vi "MAIN_test.vi"() -> ()   [LabVIEW 2016]
uses:
  <vilib>/Utility/file.llb/Write Delimited Spreadsheet (I64).vi
  BT-Android_AE_library/BT-Android_interface.lvlib
panel:
  out "String":string
  in  "Tab Control 2":enum32{"Information", "Console", "验证sd数据"}(tab)
  in  "receive frequence":i32=10
  in  "receive存盘":bool
  in  "receive file path (dialog if empty)":path=path "D:/Data/intan"
  in  "port number":u32=4321
  in  "display file path (dialog if empty)":path=path "D:/Data/intan"
  in  "display存盘":bool
  in  "Right cycle":i32
  in  "Error cycle":i32
  out "Average Error Ratio":dbl format="%#.4f"
  in  "Select IP before run":refnum<visa-resource-name>="192.168.4.1"
  in  "Channels":i32=35
  in  "START CONVERT":bool
  in  "END CONVERT":bool
  in  "校验误码率":bool
  in  "35channel存sd卡":bool
  in  "sd file path":path=path "D:/Data/intan"
  in  "验证sd数据":bool
  in  "Tab Control":enum32{"Page 1", "Page 2"}(tab)
  out "校验Array":u8[](array[numeric])
  out "高8位Array":u8[](array[numeric])
  out "低8位Array":u8[](array[numeric])
  out "display array":u16[](array[numeric])
  out "35通道波形":u16[][](graph)
  out "End Character?":bool
  out "send timeout":bool=TRUE
  out "?":bool=TRUE
  in  "convert?":bool=TRUE
  in  "Send":bool
  in  "Receive":bool=TRUE
  in  "Data Send":string
  out "error out":errorcluster
  in  "Close Com":bool
  in  "timeout (10sec)":u32=10000
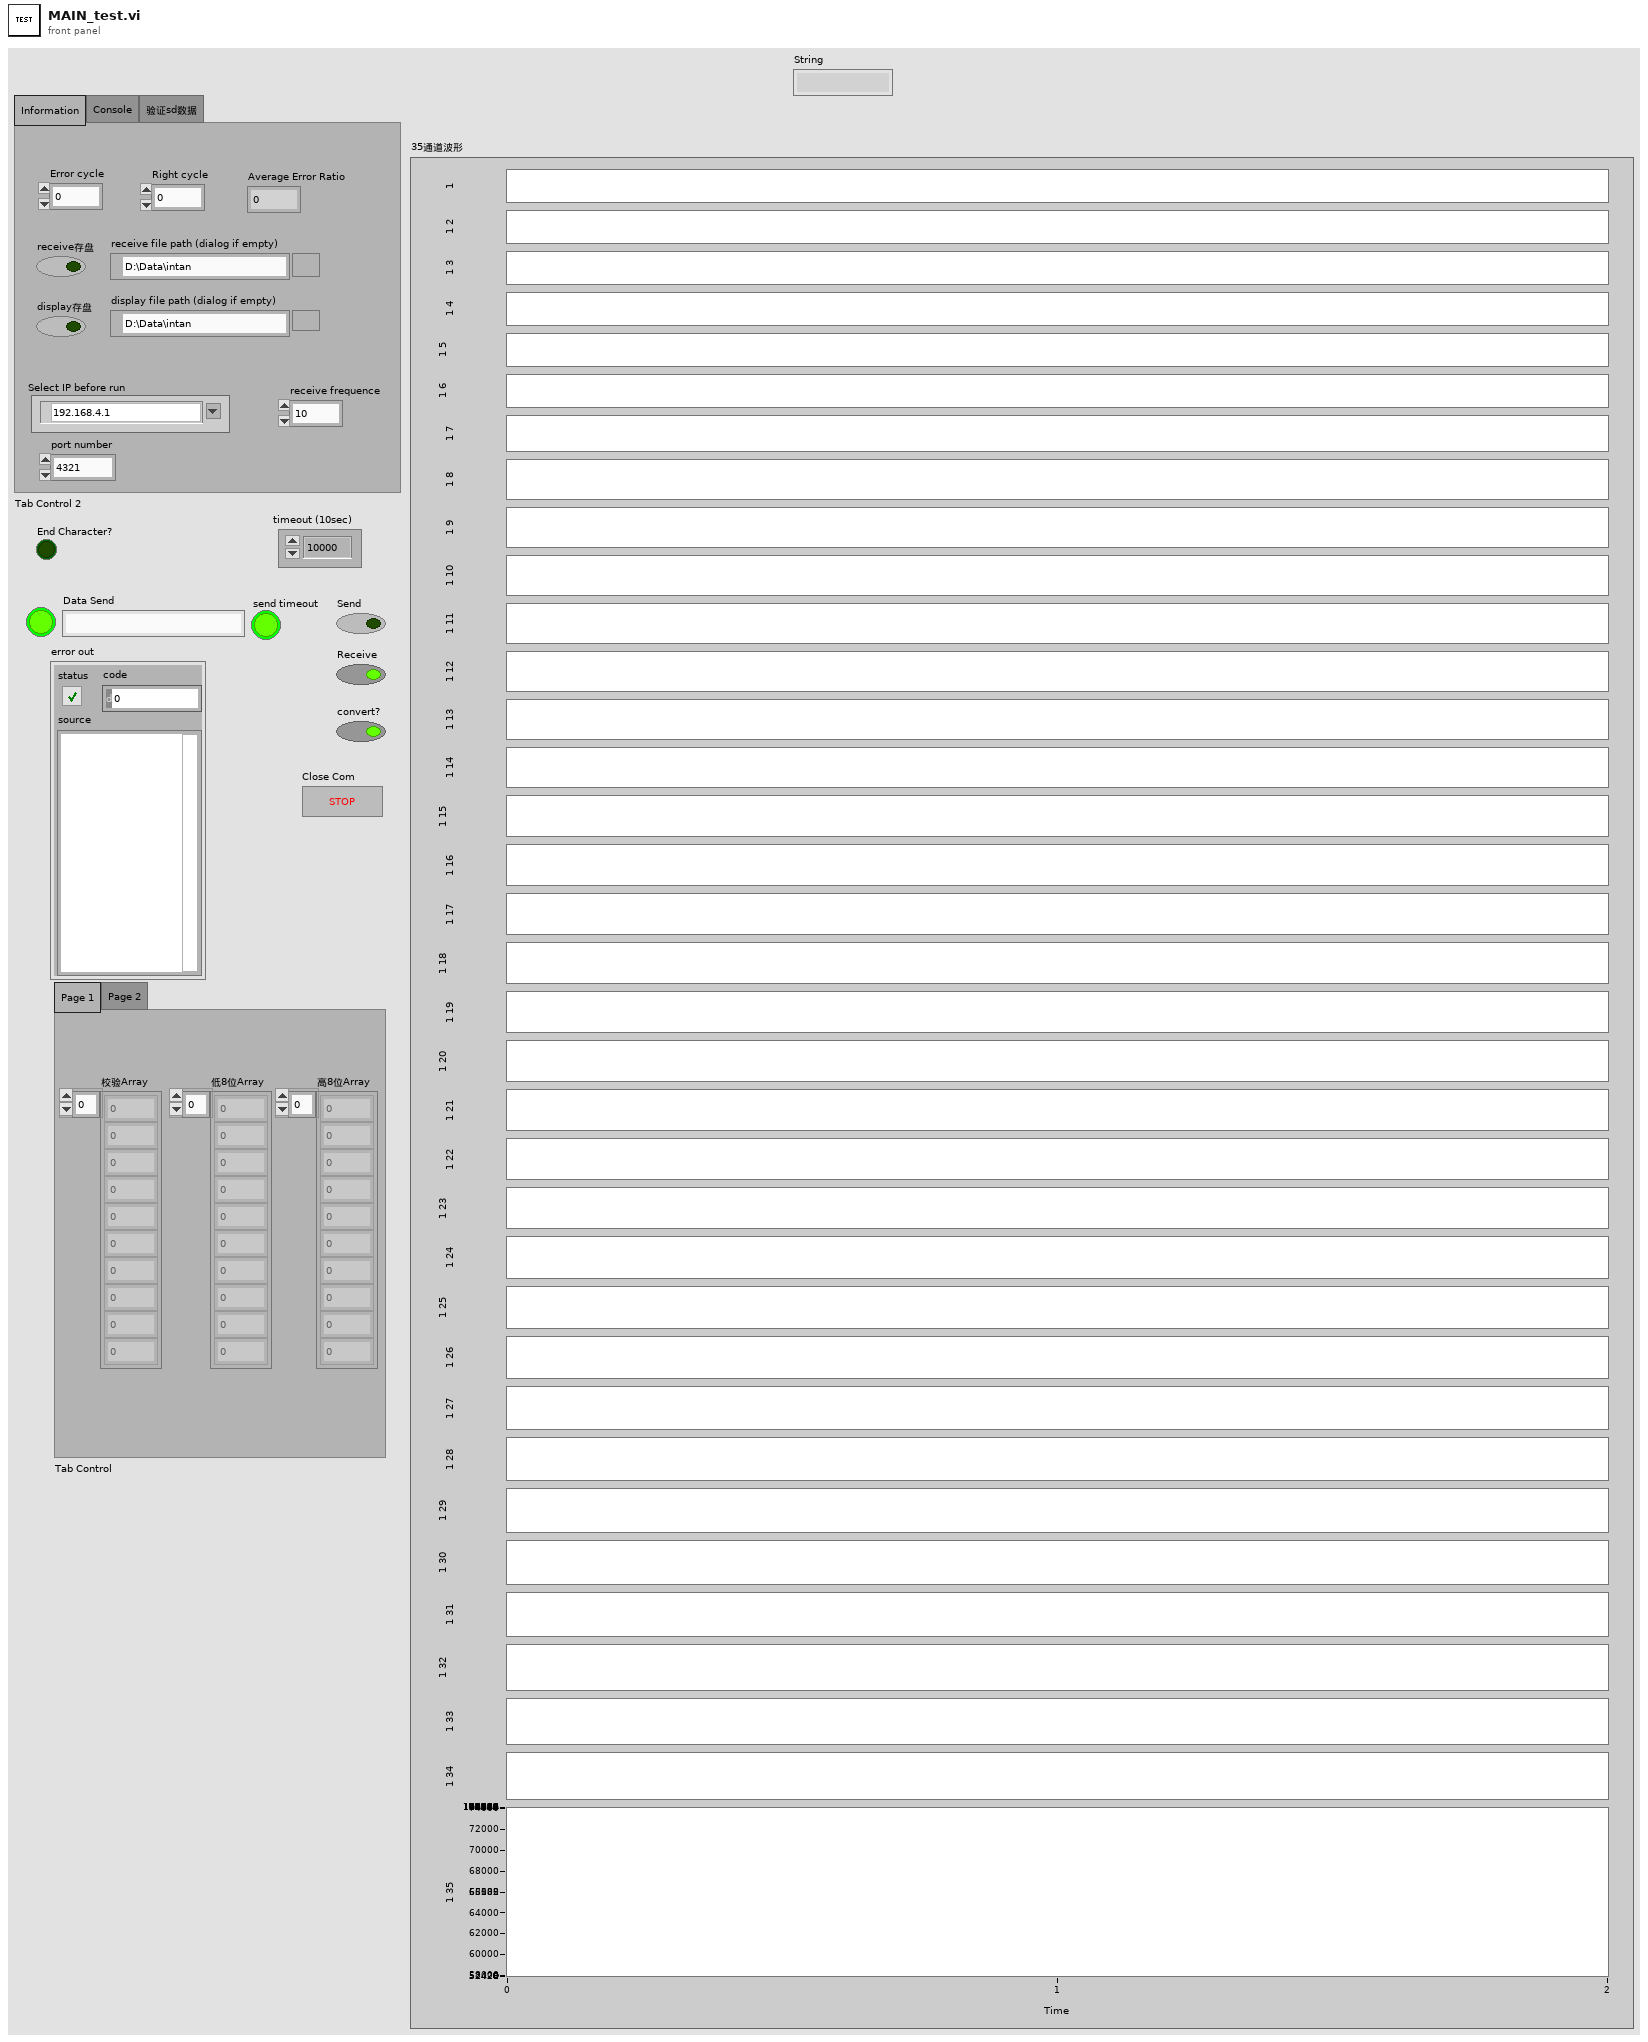
[diagram p1: front panel]
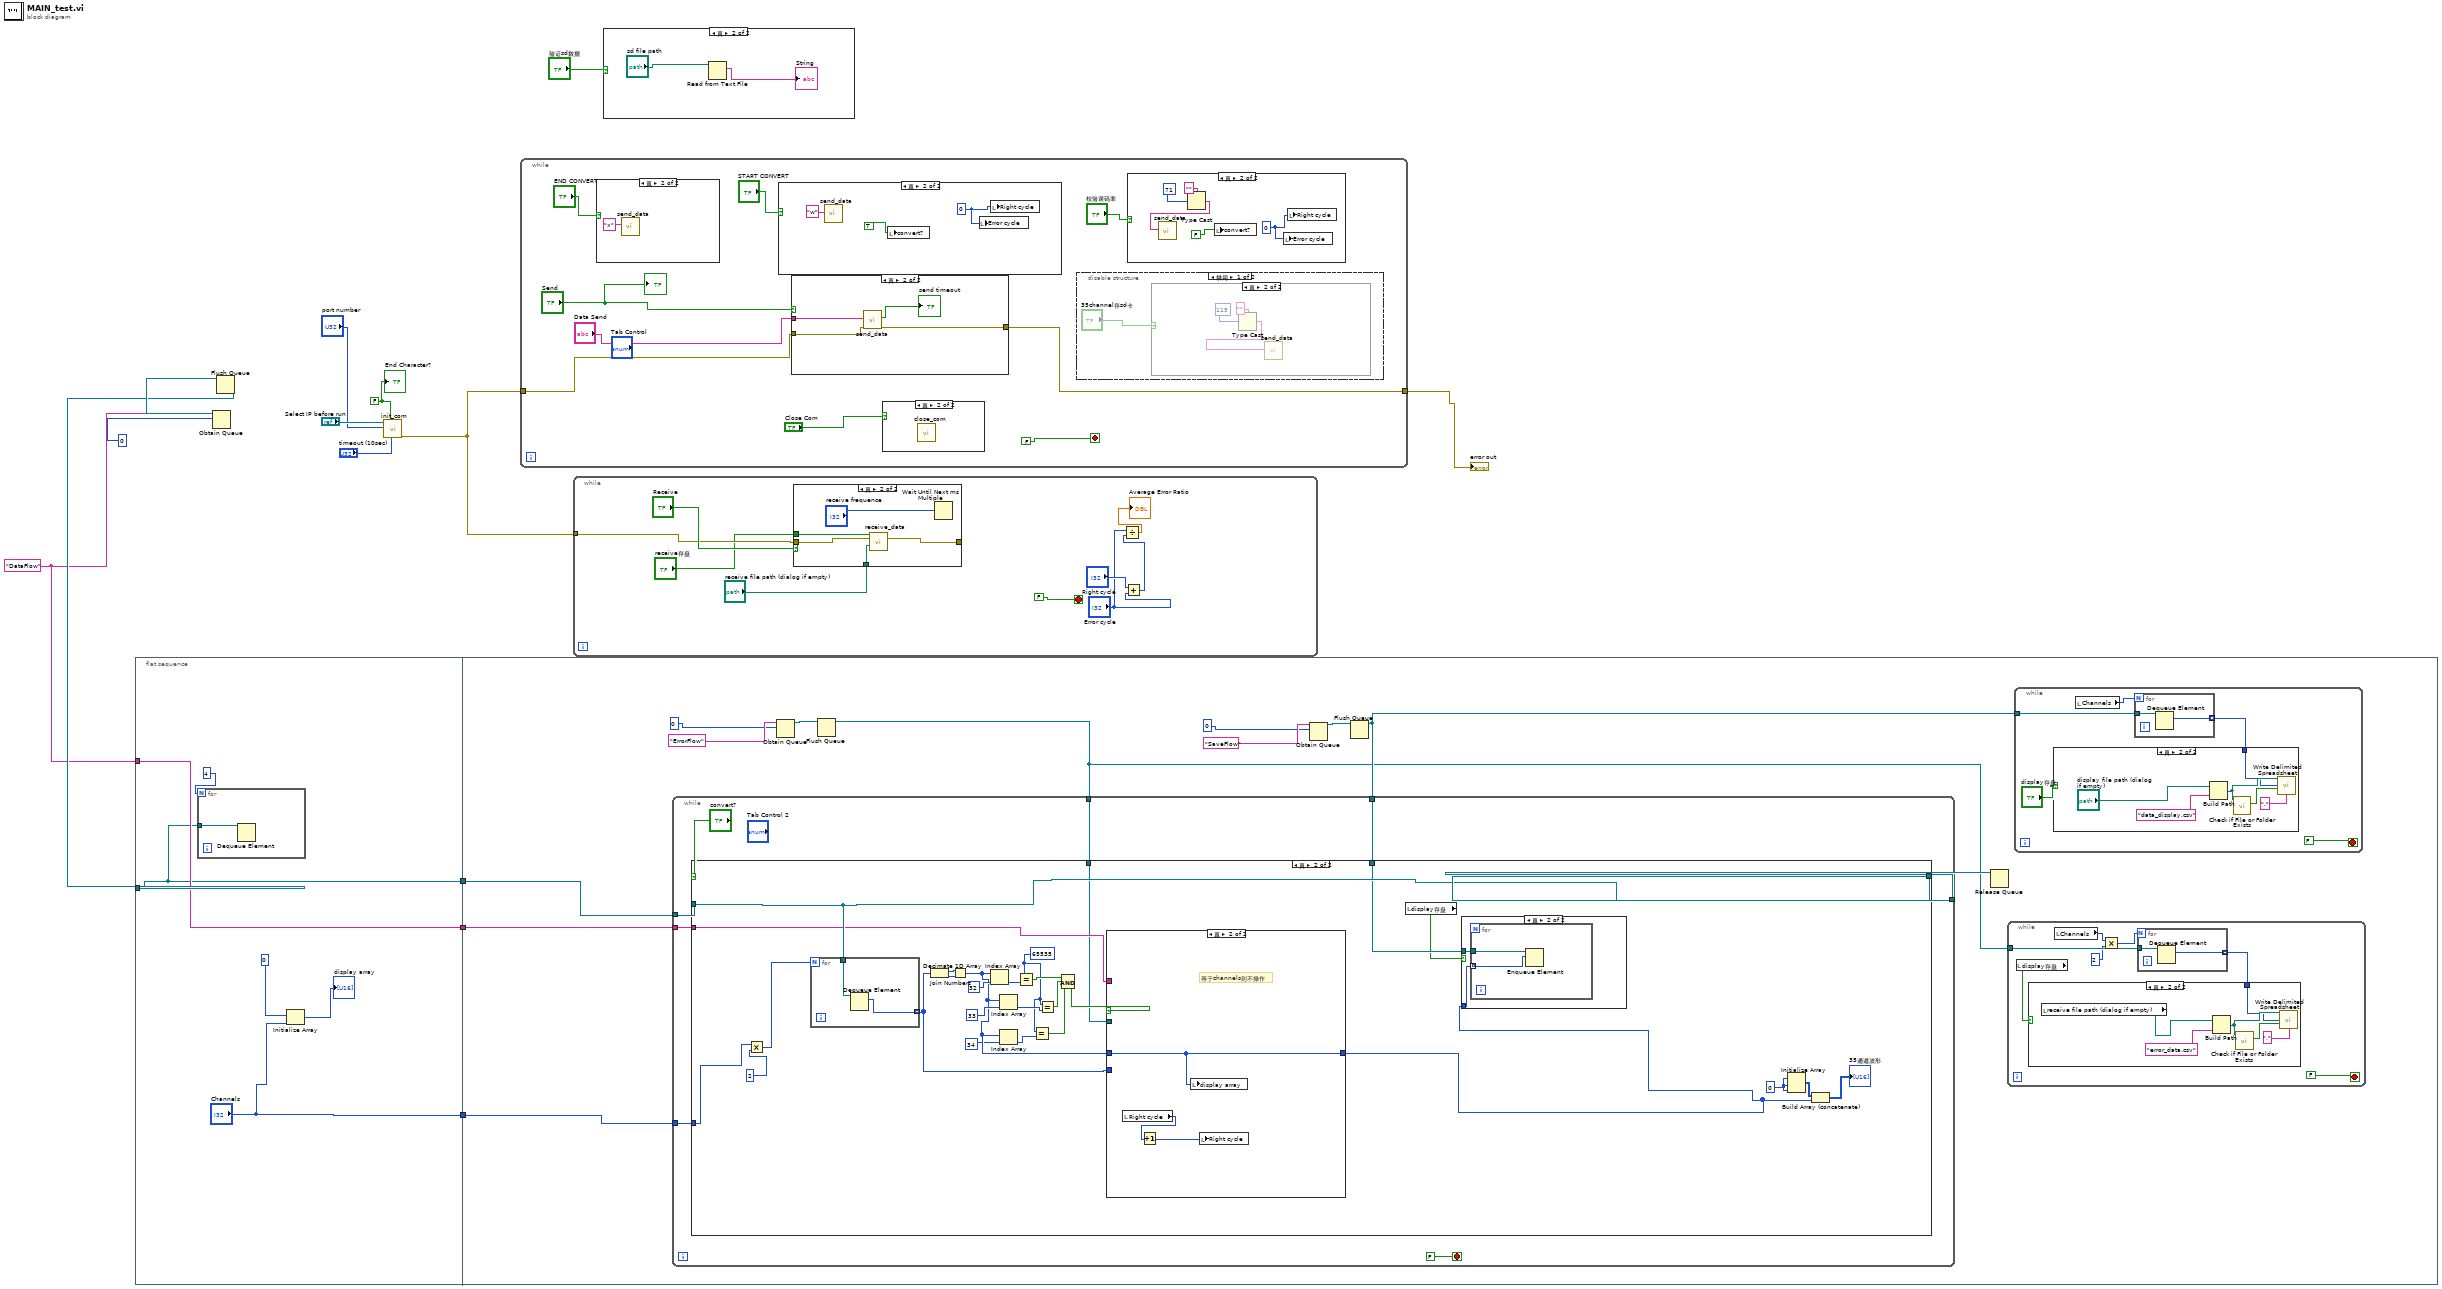
[diagram p0: block diagram]
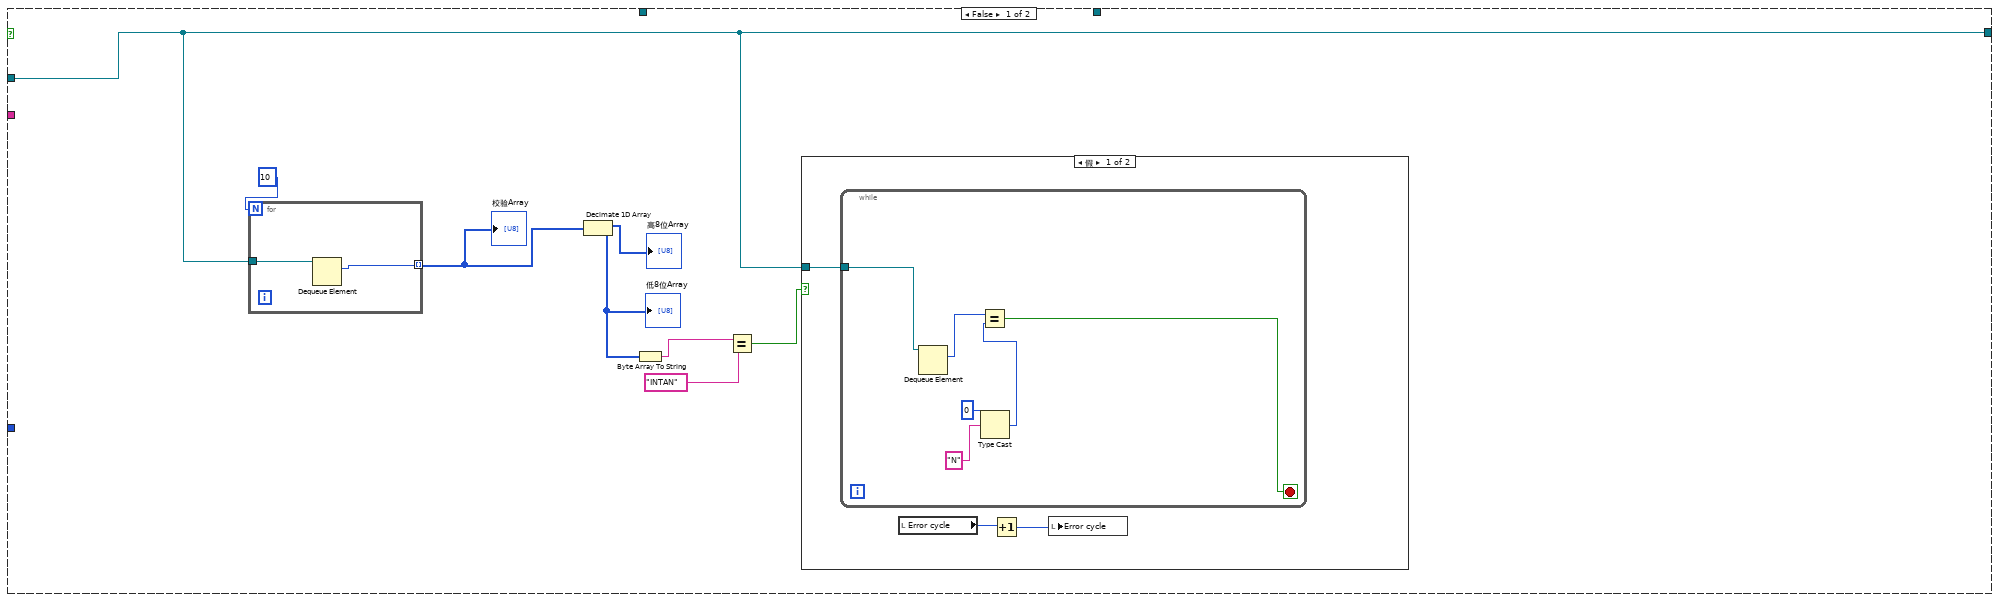
[diagram p5: hidden frame]
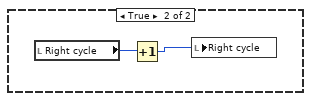
[diagram p6: hidden frame]
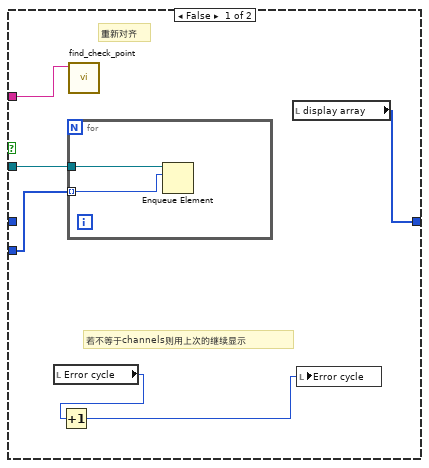
[diagram p8: hidden frame]
diagram:
  w4 = "DataFlow" ("name (unnamed)")
  w9 = FALSE ("End Write on Termination Character?")
  n1 = flat-sequence {
    tunnel: w7 -> [w16]
    tunnel: [w16] -> w6
    tunnel: w4 -> [w20]
    tunnel: [w20] -> w3
    tunnel: ["Channels"] -> w2
    tunnel: w6 -> [w33]
    tunnel: w3 -> [w32]
    tunnel: w2 -> [w31]
    frame #0 {
      n2 = for {
        N: 4 -> [_]
        tunnel: w16 -> [w21]
        n3 = Dequeue Element(queue=w21) -> ()  [unwired: 2 in, 4 out]
      }
      n4 = Initialize Array(u16 0, "Channels") -> (→"display array":u16[])
    }
    frame #1 {
      n5 = Obtain Queue(name (unnamed)="ErrorFlow", element data type=u8 0) -> (queue out=w23:refnum<queue>)  [unwired: 3 in, 2 out]
      n6 = Flush Queue(queue=w23) -> (queue out=w22:refnum<queue>)  [unwired: 1 in, 2 out]
      n7 = Obtain Queue(name (unnamed)="SaveFlow", element data type=u16 0) -> (queue out=w27:refnum<queue>)  [unwired: 3 in, 2 out]
      n8 = Flush Queue(queue=w27) -> (queue out=w26:refnum<queue>)  [unwired: 1 in, 2 out]
      n9 = while {
        tunnel: w33 -> [w68]
        tunnel: [w67] -> w30
        tunnel: w31 -> [w65]
        tunnel: w32 -> [w64]
        tunnel: w26 -> [w63]
        tunnel: w22 -> [w62]
        stop <- FALSE ("End Write on Termination Character?") stop-if-true
        n10 = case shown="真" "convert?" {
          tunnel: w68 -> [w70 w117]
          tunnel: [w70 w117] -> w67
          tunnel: w65 -> [_ w116]
          tunnel: w64 -> [_ w104]
          tunnel: w63 -> [_ w102]
          tunnel: w62 -> [_ w100]
          frame False {
            n11 = for {
              N: 10 -> [_]
              tunnel: [w90] -> w76 mode=indexing
              tunnel: w70 -> [w89]
              n12 = Dequeue Element(queue=w89) -> (element=w90:u8)  [unwired: 2 in, 3 out]
            }
            "校验Array" <- w76
            n13 = Decimate 1D Array(w76) -> (→"高8位Array":u8[], w74:u8[])
            "低8位Array" <- w74
            n14 = Byte Array To String(unsigned byte array=w74) -> (string=w73:string)
            n15 = Equal?(x=w73, y="INTAN") -> (x = y?=w71:bool)
            n16 = case shown="假" w71 {
              tunnel: w70 -> [w78 _]
              frame False {
                n17 = while {
                  tunnel: w78 -> [w86]
                  stop <- w81 stop-if-true
                  n18 = Dequeue Element(queue=w86) -> (element=w82:u8)  [unwired: 2 in, 3 out]
                  n19 = Type Cast(type=u8 0, x="N") -> (*(type *) &x=w83:u8)
                  n20 = Equal?(x=w82, y=w83) -> (x = y?=w81:bool)
                }
                n21 = local read "Error cycle"() -> (w80:i32)
                n22 = Increment(x=w80) -> (x+1=w79:i32)
                n23 = local write "Error cycle"(w79) -> ()
              }
              frame True {
                n24 = local read "Right cycle"() -> (w88:i32)
                n25 = Increment(x=w88) -> (x+1=w87:i32)
                n26 = local write "Right cycle"(w87) -> ()
              }
            }
          }
          frame True {
            w109 = u16 0
            w92 = u16 65535
            n27 = Multiply(x=w116, y=2) -> (x*y=w114:i32)
            n28 = for {
              N: w114 -> [_]
              tunnel: w117 -> [w134]
              tunnel: [w133] -> w99 mode=indexing
              n29 = Dequeue Element(queue=w134) -> (element=w133:u8)  [unwired: 2 in, 3 out]
            }
            n30 = Decimate 1D Array(w99) -> (w113:u8[], w112:u8[])
            n31 = Join Numbers(hi=w113, lo=w112) -> ((hi.lo)=w95:u16[])
            n32 = Index Array(array=w95, index=32) -> (element=w107:u16)
            n33 = Index Array(array=w95, index=33) -> (element=w97:u16)
            n34 = Index Array(array=w95, index=34) -> (element=w93:u16)
            n35 = Equal?(x=w92, y=w107) -> (x = y?=w106:bool)
            n36 = Equal?(x=w92, y=w93) -> (x = y?=w91:bool)
            n37 = Equal?(x=w92, y=w97) -> (x = y?=w96:bool)
            n38 = Compound Arithmetic op=AND(w106, w96, w91) -> (w105:bool)
            n39 = case shown="真" w105 {
              tunnel: [w126 w132] -> w103
              tunnel: w95 -> [_ w132]
              tunnel: w104 -> [w127 _]
              tunnel: w100 -> [w125 _]
              tunnel: w99 -> [w124 _]
              frame False {
                # "重新对齐"
                # "若不等于channels则用上次的继续显示"
                n40 = local read "Error cycle"() -> (w123:i32)
                n41 = Increment(x=w123) -> (x+1=w122:i32)
                n42 = for {
                  tunnel: w124 -> [w129] mode=indexing
                  tunnel: w125 -> [w128]
                  n43 = Enqueue Element(queue=w128, element=w129) -> ()  [unwired: 2 in, 3 out]
                }
                n44 = call "find_check_point.vi"("input queue"=w127) -> ()  [unwired: 11 in]
                n45 = local read "display array"() -> (w126:u16[])
                n46 = local write "Error cycle"(w122) -> ()
              }
              frame True {
                # "等于channels则不操作"
                n47 = local read "Right cycle"() -> (w131:i32)
                n48 = Increment(x=w131) -> (x+1=w130:i32)
                n49 = local write "display array"(w132) -> ()
                n50 = local write "Right cycle"(w130) -> ()
              }
            }
            n51 = local read "display存盘"() -> (w101:bool)
            n52 = case shown="真" w101 {
              tunnel: w103 -> [_ w119]
              tunnel: w102 -> [_ w118]
              frame False {
              }
              frame True {
                n53 = for {
                  tunnel: w119 -> [w121] mode=indexing
                  tunnel: w118 -> [w120]
                  n54 = Enqueue Element(queue=w120, element=w121) -> ()  [unwired: 2 in, 3 out]
                }
              }
            }
            n55 = Initialize Array(w109, w109, w109) -> (w110:u16[][])
            n56 = Build Array (concatenate)(w110, w103) -> (→"35通道波形":u16[][])
          }
        }
      }
      n57 = Release Queue(queue=w30) -> ()  [unwired: 2 in, 3 out]
      n58 = while {
        tunnel: w22 -> [w39]
        stop <- FALSE stop-if-true
        n59 = local read "display存盘"() -> (w37:bool)
        n60 = local read "Channels"() -> (w35:i32)
        n61 = Multiply(x=w35, y=2) -> (x*y=w34:i32)
        n62 = for {
          N: w34 -> [_]
          tunnel: w39 -> [w42]
          tunnel: [w41] -> w38 mode=indexing
          n63 = Dequeue Element(queue=w42) -> (element=w41:u8)  [unwired: 2 in, 3 out]
        }
        n64 = case shown="真" w37 {
          tunnel: w38 -> [_ w44]
          frame False {
          }
          frame True {
            n65 = local read "receive file path (dialog if empty)"() -> (w43:path)
            n66 = Build Path(base path=w43, name or relative path="error_data.csv") -> (appended path=w48:path)
            n67 = call <vilib>:"Check if File or Folder Exists.vi"("path"=w48) -> ("file or folder exists?"=w47:bool)  [unwired: 8 in, 2 out]
            n68 = call-poly <vilib>:"Write Delimited Spreadsheet.vi"("file path (dialog if empty)"=w48, "1D data"=w44, "append to file? (new file:F)"=w47, "delimiter (\\t)"="," ("delimiter (\\t)")) -> ()  [unwired: 10 in, 2 out]
          }
        }
      }
      n69 = while {
        tunnel: w26 -> [w50]
        stop <- FALSE stop-if-true
        n70 = local read "Channels"() -> (w51:i32)
        n71 = for {
          N: w51 -> [_]
          tunnel: w50 -> [w55]
          tunnel: [w54] -> w49 mode=indexing
          n72 = Dequeue Element(queue=w55) -> (element=w54:u16)  [unwired: 2 in, 3 out]
        }
        n73 = case shown="真" "display存盘" {
          tunnel: w49 -> [_ w56]
          frame False {
          }
          frame True {
            n74 = Build Path(base path="display file path (dialog if empty)", name or relative path="data_display.csv") -> (appended path=w61:path)
            n75 = call <vilib>:"Check if File or Folder Exists.vi"("path"=w61) -> ("file or folder exists?"=w60:bool)  [unwired: 8 in, 2 out]
            n76 = call-poly <vilib>:"Write Delimited Spreadsheet.vi"("file path (dialog if empty)"=w61, "1D data"=w56, "append to file? (new file:F)"=w60, "delimiter (\\t)"="," ("delimiter (\\t)")) -> ()  [unwired: 10 in, 2 out]
          }
        }
      }
    }
  }
  n77 = Obtain Queue(name (unnamed)=w4, element data type=u8 0) -> (queue out=w10:refnum<queue>)  [unwired: 3 in, 2 out]
  n78 = Flush Queue(queue=w10) -> (queue out=w7:refnum<queue>)  [unwired: 1 in, 2 out]
  n79 = call "init_com.vi"("timeout (10sec)"="timeout (10sec)", "End Write on Termination Character?"=w9, "port"="port number", "VISA resource name"="Select IP before run") -> ("error out"=w11:errorcluster)  [unwired: 7 in]
  n80 = while {
    tunnel: w11 -> [w141]
    tunnel: [w142] -> w8
    stop <- FALSE ("End Write on Termination Character?") stop-if-true
    n81 = case shown="真" "END CONVERT" {
      frame False {
      }
      frame True {
        n82 = call "send_data.vi"("send data (string)"="x") -> ()  [unwired: 9 in, 2 out]
      }
    }
    n83 = case shown="真" "START CONVERT" {
      frame False {
      }
      frame True {
        w155 = 0
        n84 = call "send_data.vi"("send data (string)"="w") -> ()  [unwired: 9 in, 2 out]
        n85 = local write "convert?"(TRUE) -> ()
        n86 = local write "Error cycle"(w155) -> ()
        n87 = local write "Right cycle"(w155) -> ()
      }
    }
    n88 = case shown="真" "Send" {
      tunnel: "Data Send" -> [_ w161]
      tunnel: w141 -> [w157 w160]
      tunnel: [w157 w159] -> w142
      frame False {
      }
      frame True {
        n89 = call "send_data.vi"("error in (no error)"=w160, "send data (string)"=w161) -> ("error out"=w159:errorcluster, "timeout?"=→"send timeout":bool)  [unwired: 8 in]
      }
    }
    n90 = case shown="真" "Close Com" {
      frame False {
      }
      frame True {
        n91 = call "close_com.vi"() -> ()  [unwired: 11 in, 1 out]
      }
    }
    n92 = disable-structure shown="禁用" {
      frame Disabled {
        n93 = case shown="真" "35channel存sd卡" {
          frame False {
          }
          frame True {
            n94 = Type Cast(type="" ("Data Send 2"), x=115) -> (*(type *) &x=w145:string)
            n95 = call "send_data.vi"("send data (string)"=w145) -> ()  [unwired: 9 in, 2 out]
          }
        }
      }
      frame Enabled {
      }
    }
    n96 = case shown="真" "校验误码率" {
      frame False {
      }
      frame True {
        w151 = 0
        n97 = Type Cast(type="" ("Data Send 2"), x=71) -> (*(type *) &x=w148:string)
        n98 = call "send_data.vi"("send data (string)"=w148) -> ()  [unwired: 9 in, 2 out]
        n99 = local write "convert?"(FALSE) -> ()
        n100 = local write "Error cycle"(w151) -> ()
        n101 = local write "Right cycle"(w151) -> ()
      }
    }
    "?" <- "Send"
  }
  "error out" <- w8
  n102 = while {
    tunnel: w11 -> [w169]
    stop <- FALSE ("End Write on Termination Character?") stop-if-true
    n103 = case shown="真" "Receive" {
      tunnel: w169 -> [w171 w175]
      tunnel: [w171 w174] -> _
      tunnel: "receive存盘" -> [_ w173]
      tunnel: "receive file path (dialog if empty)" -> [_ w172]
      frame False {
      }
      frame True {
        n104 = call "receive_data.vi"("存盘"=w173, "error in (no error)"=w175, "file path (dialog if empty)"=w172) -> ("error out"=w174:errorcluster)  [unwired: 11 in, 1 out]
        n105 = Wait Until Next ms Multiple(millisecond multiple="receive frequence") -> ()  [unwired: 1 out]
      }
    }
    n106 = Add(x="Right cycle", y="Error cycle") -> (x+y=w163:i32)
    n107 = Divide(x="Error cycle", y=w163) -> (x/y=→"Average Error Ratio":dbl)
  }
  n108 = case shown="真" "验证sd数据" {
    frame False {
    }
    frame True {
      n109 = Read from Text File(file (use dialog)="sd file path") -> (text=→"String":string)  [unwired: 3 in, 3 out]
    }
  }
  "End Character?" <- w9
